vi "Create Channel.vi"(8 "error in (no error)":errorcluster, 9 "Resource (None)":string, 10 "Name":string, 11 "Group in":refnum<class "Group Config.lvclass">) -> (0 "error out":errorcluster, 2 "Channel":refnum<class "Channel Config.lvclass">, 3 "Group out":refnum<class "Group Config.lvclass">)   [LabVIEW 2020, in "VolatusConfig.lvlib" / "Group Config.lvclass"]
uses:
  Group Config.lvclass
  Group Config.lvclass/Group Config.ctl
  VolatusConfigElement/VolatusConfigElement.lvclass
  Channel/Channel Config.lvclass
  C:/dev/lv20CE/relink/lv-volatus/VolatusConfig/VolatusConfigElement/VolatusConfigElement.lvclass
  C:/dev/lv20CE/relink/lv-volatus/VolatusConfig/Group/Group Config.lvclass
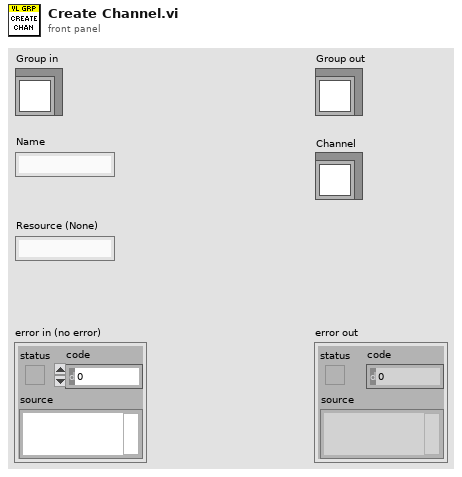
[diagram p1: front panel]
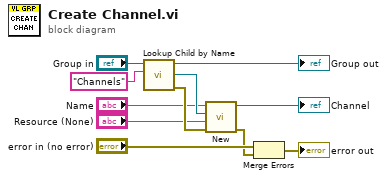
[diagram p0: block diagram]
diagram:
  n1 = call "Lookup Child by Name.vi"("Child Name"="Channels", "VolatusConfigElement in"="Group in") -> ("error out"=w11:errorcluster, "Child"=w6:refnum<class "Config Element.lvclass">, "VolatusConfigElement out"=→"Group out":refnum<class "Group Config.lvclass">)  [unwired: 6 in, 1 out]
  n2 = call "New.vi"("error in (no error)"=w11, "Resource (None)"="Resource (None)", "Parent"=w6, "Name"="Name") -> ("error out"=w2:errorcluster, "Channel out"=→"Channel":refnum<class "Channel Config.lvclass">)  [unwired: 6 in]
  n3 = Merge Errors("error in (no error)", w2) -> (→"error out":errorcluster)
